vi "Scrape WPC Financial Stats.vi"() -> (0 "error out":errorcluster, 1 "redacted?":bool, 2 "WPC Financial Cash Stats":cluster{"Player":string, "Cash Profit":dbl}[](array[cluster]), 3 "WPC Financial Tournament Stats":T1(array[cluster]))   [LabVIEW 2021]
uses:
  <vilib>/httpClient/LabVIEWHTTPClient.lvlib
panel:
  out "body":string
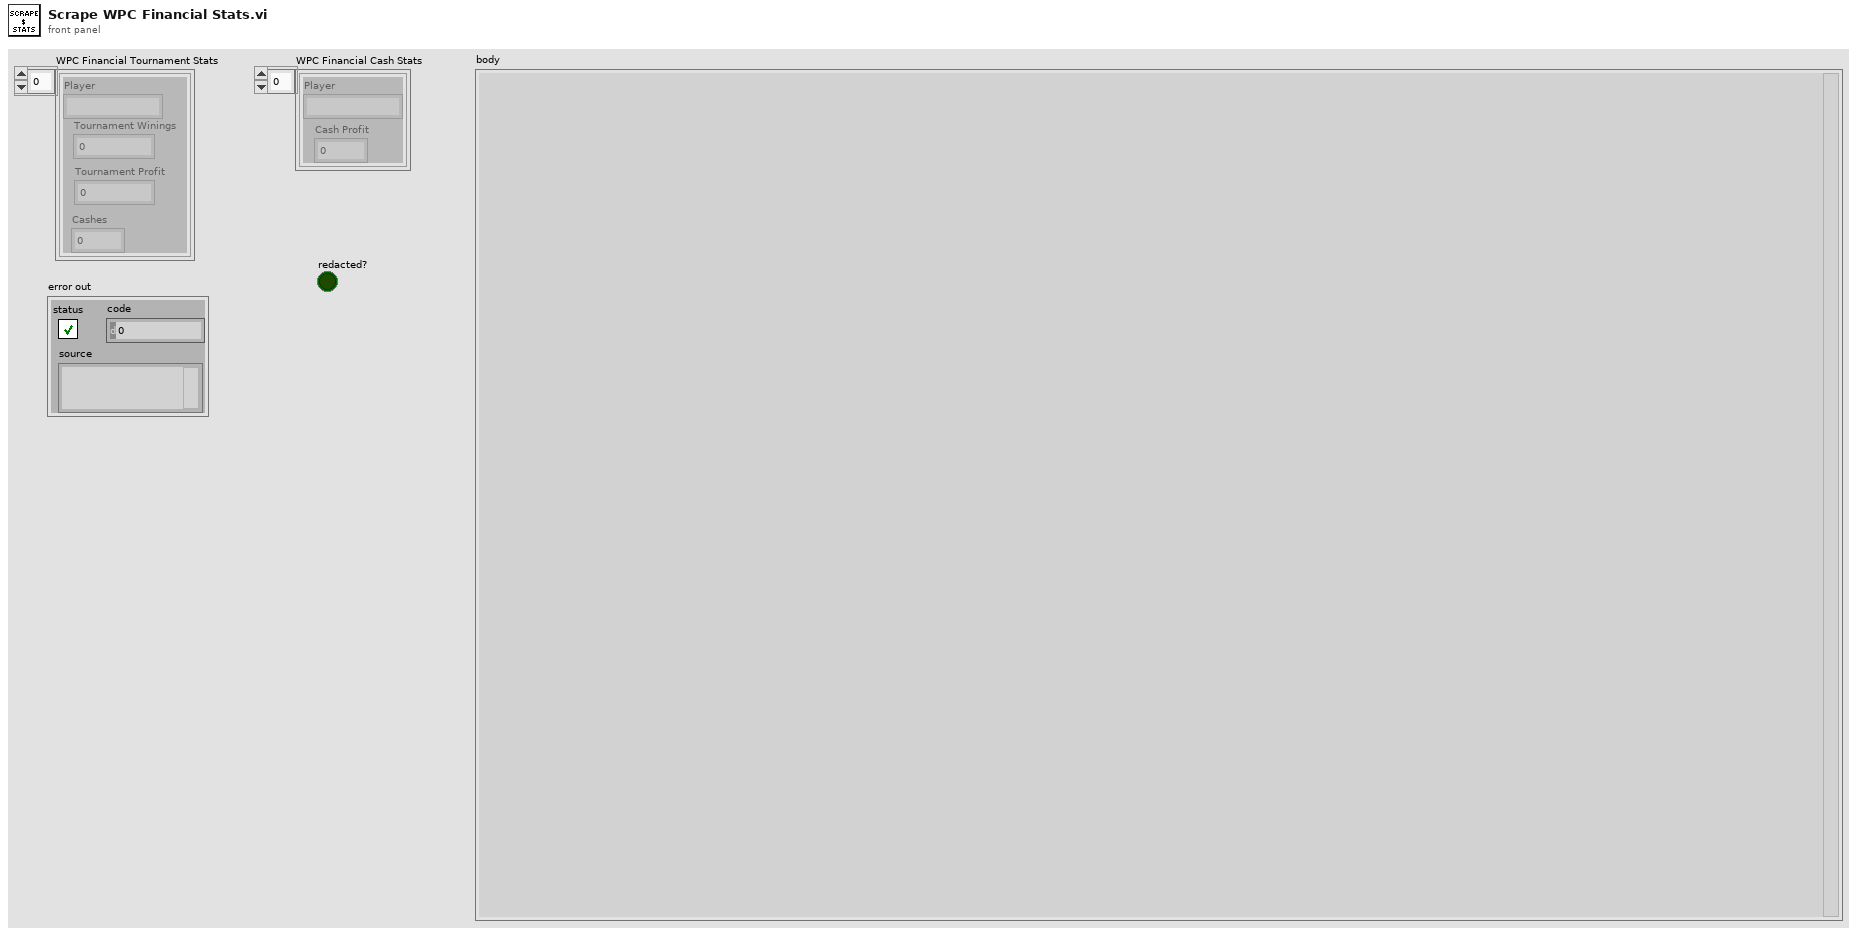
[diagram p1: front panel]
types:
  T1 = cluster{"Player":string, "Tournament Winings":dbl, "Tournament Profit":dbl, "Cashes":dbl}[]
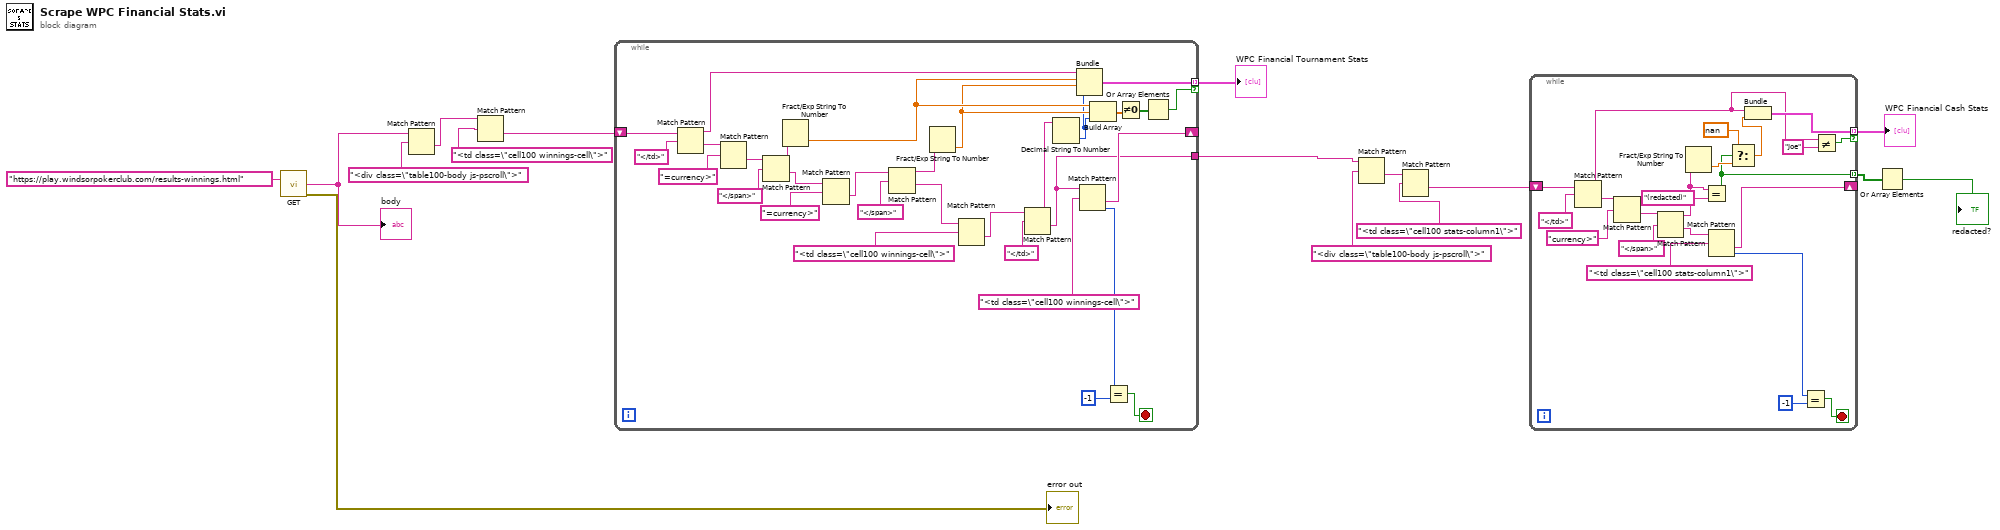
[diagram p0: block diagram]
diagram:
  n1 = call <vilib>:"GET.vi"("url"="https://play.windsorpokerclub.com/results-winnings.html") -> ("body"=w14:string, "error out"=→"error out":errorcluster)  [unwired: 11 in, 2 out]
  "body" <- w14
  n2 = Match Pattern(string=w14, regular expression="<div class=\"table100-body js-pscroll\">") -> (after substring=w12:string)  [unwired: 1 in, 3 out]
  n3 = Match Pattern(string=w12, regular expression="<td class=\"cell100 winnings-cell\">") -> (after substring=w10:string)  [unwired: 1 in, 3 out]
  n4 = while {
    shift-right: [w26] -> _
    shift-left: w10 -> [w47]
    tunnel: [w35] -> w3 mode=indexing if=w17
    tunnel: [w24] -> w9
    stop <- w38 stop-if-true
    n5 = Match Pattern(string=w47, regular expression="</td>") -> (before substring=w37:string, after substring=w45:string)  [unwired: 1 in, 2 out]
    n6 = Match Pattern(string=w45, regular expression="=currency>") -> (after substring=w43:string)  [unwired: 1 in, 3 out]
    n7 = Match Pattern(string=w43, regular expression="</span>") -> (before substring=w34:string, after substring=w33:string)  [unwired: 1 in, 2 out]
    n8 = Fract/Exp String To Number(string=w34) -> (number=w22:dbl)  [unwired: 3 in, 1 out]
    n9 = Match Pattern(string=w33, regular expression="=currency>") -> (after substring=w31:string)  [unwired: 1 in, 3 out]
    n10 = Match Pattern(string=w31, regular expression="</span>") -> (before substring=w36:string, after substring=w28:string)  [unwired: 1 in, 2 out]
    n11 = Fract/Exp String To Number(string=w36) -> (number=w21:dbl)  [unwired: 3 in, 1 out]
    n12 = Match Pattern(string=w28, regular expression="<td class=\"cell100 winnings-cell\">") -> (after substring=w29:string)  [unwired: 1 in, 3 out]
    n13 = Match Pattern(string=w29, regular expression="</td>") -> (before substring=w23:string, after substring=w24:string)  [unwired: 1 in, 2 out]
    n14 = Decimal String To Number(string=w23) -> (number=w20:i32)  [unwired: 2 in, 1 out]
    n15 = Bundle("body"=w37, w22, w21, w20) -> (w35:cluster{"body":string, dbl, dbl, i32})  [unwired: 1 in]
    n16 = Match Pattern(string=w24, regular expression="<td class=\"cell100 winnings-cell\">") -> (after substring=w26:string, offset past match=w40:i32)  [unwired: 1 in, 2 out]
    n17 = Build Array(w22, w21, w20) -> (w19:dbl[])
    n18 = Equal?(x=w40, y=-1) -> (x = y?=w38:bool)
    n19 = Not Equal To 0?(x=w19) -> (x != 0?=w18:bool[])
    n20 = Or Array Elements(Boolean array=w18) -> (logical OR=w17:bool)
  }
  "WPC Financial Tournament Stats" <- w3
  n21 = Match Pattern(string=w9, regular expression="<div class=\"table100-body js-pscroll\">") -> (after substring=w7:string)  [unwired: 1 in, 3 out]
  n22 = Match Pattern(string=w7, regular expression="<td class=\"cell100 stats-column1\">") -> (after substring=w5:string)  [unwired: 1 in, 3 out]
  n23 = while {
    shift-right: [w61] -> _
    shift-left: w5 -> [w69]
    tunnel: [w57] -> w4 mode=indexing if=w50
    tunnel: [w51] -> w2 mode=indexing
    stop <- w59 stop-if-true
    n24 = Match Pattern(string=w69, regular expression="</td>") -> (before substring=w49:string, after substring=w67:string)  [unwired: 1 in, 2 out]
    n25 = Match Pattern(string=w67, regular expression="currency>") -> (after substring=w65:string)  [unwired: 1 in, 3 out]
    n26 = Match Pattern(string=w65, regular expression="</span>") -> (before substring=w56:string, after substring=w63:string)  [unwired: 1 in, 2 out]
    n27 = Fract/Exp String To Number(string=w56) -> (number=w54:dbl)  [unwired: 3 in, 1 out]
    n28 = Equal?(x=w56, y="(redacted)") -> (x = y?=w51:bool)
    n29 = Match Pattern(string=w63, regular expression="<td class=\"cell100 stats-column1\">") -> (after substring=w61:string, offset past match=w58:i32)  [unwired: 1 in, 2 out]
    n30 = Select(t=nan, s=w51, f=w54) -> (s? t:f=w53:dbl)
    n31 = Bundle("body"=w49, w53) -> (w57:cluster{"body":string, dbl})  [unwired: 1 in]
    n32 = Equal?(x=w58, y=-1) -> (x = y?=w59:bool)
    n33 = Not Equal?(x=w49, y="Joe") -> (x != y?=w50:bool)
  }
  "WPC Financial Cash Stats" <- w4
  n34 = Or Array Elements(Boolean array=w2) -> (logical OR=→"redacted?":bool)
